vi "Convert Device Units to Acceleration Units.vi"(9 "Microstep Size (0)":dbl, 10 "Units (0: device acceleration units)":u16(ring) items=["device acceleration units", "microsteps per second squared", "microns per second squared", "millimeters per second squared", "inches per second squared", "degrees per second squared"], 11 "Device Acceleration (0)":i32) -> (3 "Acceleration":dbl)   [LabVIEW 2013, in "Zaber A Series.lvlib"]
doc: "Helper to convert device-specific units of acceleration to standard units.\n\nSelect a unit and enter an a device's acceleration quantity. The output will be the acceleration converted to the selected unit.\n\nIf you select a unit other than device units, you must also provide the Microstep Size conversion factor from microsteps to micrometers, which can be found in your device manual."
uses:
  Zaber A Series.lvlib
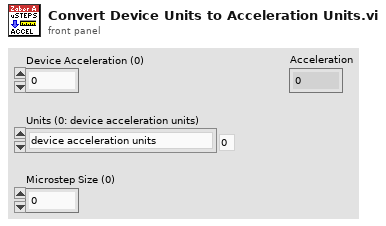
[diagram p1: front panel]
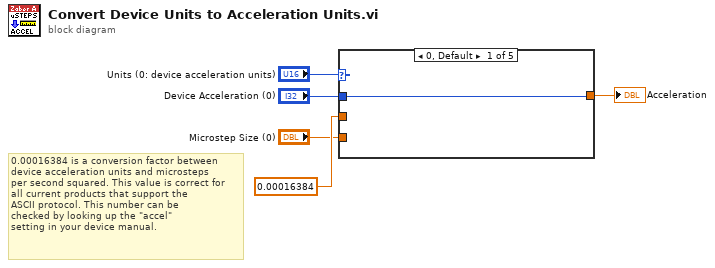
[diagram p0: block diagram]
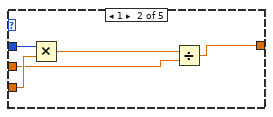
[diagram p2: hidden frame]
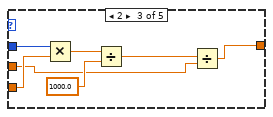
[diagram p3: hidden frame]
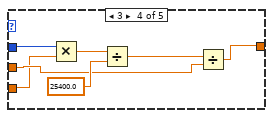
[diagram p4: hidden frame]
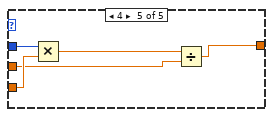
[diagram p5: hidden frame]
diagram:
  # "0.00016384 is a conversion factor between \ndevice acceleration units and microsteps \nper second squared. This value is correct for\nall current products that support the\nASCII protocol. This number can be \nchecked by looking up the \"accel\"\nsetting in your device manual."
  n1 = case shown="0, Default" "Units (0: device acceleration units)" {
    tunnel: 0.00016384 ("Acceleration Constant (0.00016384)") -> [_ w9 w14 w21 w27]
    tunnel: "Microstep Size (0)" -> [_ w10 w17 w20 w29]
    tunnel: [w6 w8 w13 w23 w28] -> w1
    tunnel: "Device Acceleration (0)" -> [w6 w11 w18 w22 w30]
    frame 0, Default {
    }
    frame 1 {
      n2 = Multiply(x=w11, y=w10) -> (x*y=w7:dbl)
      n3 = Divide(x=w7, y=w9) -> (x/y=w8:dbl)
    }
    frame 2 {
      n4 = Multiply(x=w18, y=w17) -> (x*y=w16:dbl)
      n5 = Divide(x=w16, y=1000.0) -> (x/y=w12:dbl)
      n6 = Divide(x=w12, y=w14) -> (x/y=w13:dbl)
    }
    frame 3 {
      n7 = Multiply(x=w22, y=w20) -> (x*y=w25:dbl)
      n8 = Divide(x=w25, y=25400.0) -> (x/y=w19:dbl)
      n9 = Divide(x=w19, y=w21) -> (x/y=w23:dbl)
    }
    frame 4 {
      n10 = Multiply(x=w30, y=w29) -> (x*y=w26:dbl)
      n11 = Divide(x=w26, y=w27) -> (x/y=w28:dbl)
    }
  }
  "Acceleration" <- w1
